vi "Mock MVA Caller.vi"() -> ()   [LabVIEW 2019]
panel:
  in  "bnshgds":string="sajklf;jdkas" caption="Datum Name"
  in  "Cluster 2":cluster{"Cluster":cluster{"String":string}}
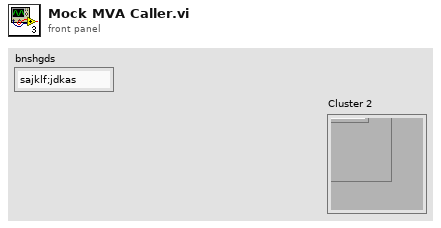
[diagram p1: front panel]
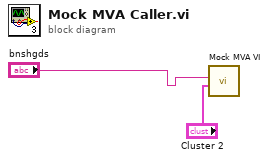
[diagram p0: block diagram]
diagram:
  n1 = call "Mock MVA VI.vi"("Datum Value"="Cluster 2", "Datum Name"="bnshgds") -> ()  [unwired: 10 in]
